vi "LV_json_read.vi"() -> ()   [LabVIEW 2020]
panel:
  out "error out":errorcluster
  out "value":T1(array[cluster])
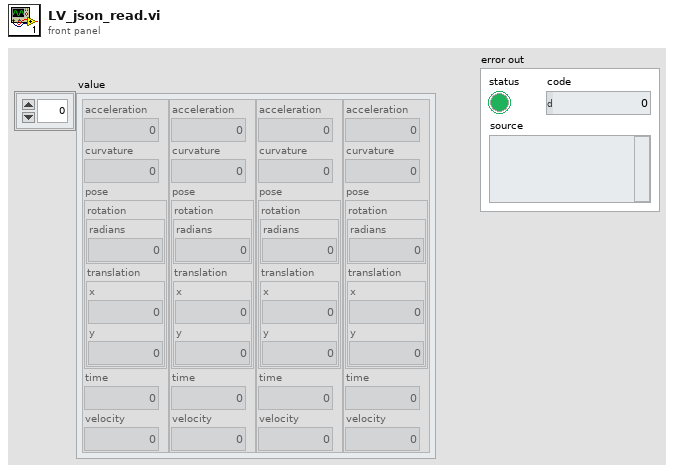
[diagram p1: front panel]
types:
  T1 = cluster{"acceleration":dbl, "curvature":dbl, "pose":cluster{"rotation":cluster{"radians":dbl}, "translation":cluster{"x":dbl, "y":dbl}}, "time":dbl, "velocity":dbl}[]
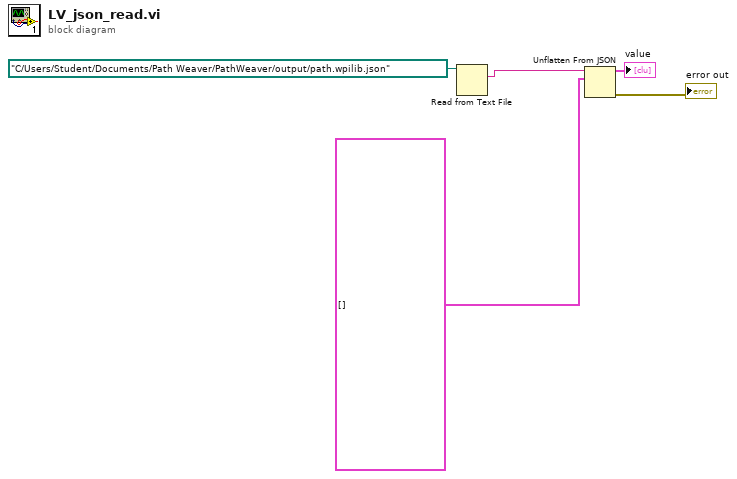
[diagram p0: block diagram]
diagram:
  n1 = Read from Text File(file (use dialog)=path "C:/Users/Student/Documents/Path Weaver/PathWeaver/output/path.wpilib.json") -> (text=w5:string)  [unwired: 3 in, 3 out]
  n2 = Unflatten From JSON(JSON string=w5, type and defaults=T1 []) -> (value=→"value":T1, error out=→"error out":errorcluster)  [unwired: 5 in]
